vi "CodeDetection(SubVI).vi"(1 "Code":dbl[](array[numeric]), 2 "Buff":dbl[](array[numeric]), 3 "L_sum":i32) -> (0 "detect":bool)   [LabVIEW 2017]
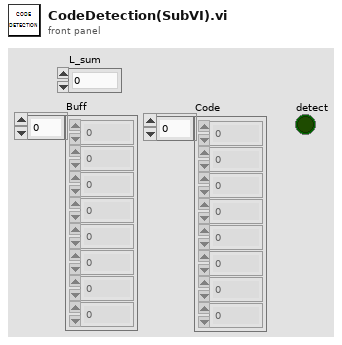
[diagram p1: front panel]
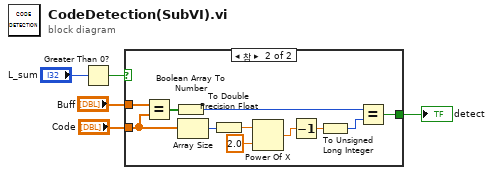
[diagram p0: block diagram]
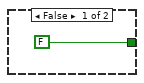
[diagram p2: hidden frame]
diagram:
  n1 = Greater Than 0?(x="L_sum") -> (x > 0?=w4:bool)
  n2 = case shown="참" w4 {
    tunnel: [FALSE w12] -> w2
    tunnel: "Code" -> [_ w14]
    tunnel: "Buff" -> [_ w15]
    frame False {
    }
    frame True {
      n3 = Equal?(x=w15, y=w14) -> (x = y?=w17:bool[])
      n4 = Boolean Array To Number(Boolean array=w17) -> (number=w16:u32)
      n5 = Array Size(array=w14) -> (size(s)=w10:i32)
      n6 = To Double Precision Float(number=w10) -> (double precision float=w9:dbl)
      n7 = Power Of X(1:2.0 ("x"), 2:w9) -> (0:w8:dbl)
      n8 = Decrement(x=w8) -> (x-1=w13:dbl)
      n9 = To Unsigned Long Integer(number=w13) -> (unsigned 32bit integer=w7:u32)
      n10 = Equal?(x=w16, y=w7) -> (x = y?=w12:bool)
    }
  }
  "detect" <- w2
